vi "绘制语法框.vi"(8 "error in":errorcluster caption="错误输入（无错误）", 11 "程序 输入":refnum<class "程序.lvclass">) -> (0 "error out":errorcluster caption="错误输出", 3 "程序 输出":refnum<class "程序.lvclass">)   [LabVIEW 2020, in "程序.lvclass"]
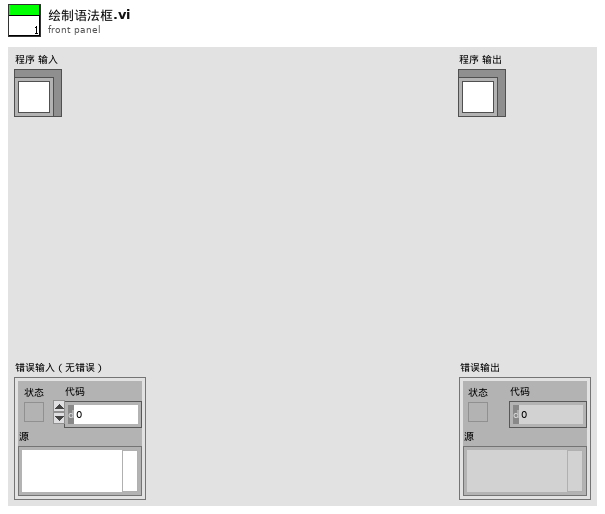
[diagram p1: front panel]
types:
  T1 = cluster{"left":i16, "top":i16, "right":i16, "bottom":i16}
  T2 = cluster{"Width":i16, "Style":enum32{"Solid", "Dash", "Dot", "DashDot", "DashDotDot"}}
  T3 = typedef "LVBoundsTypeDef.ctl" = cluster{"Width":u32, "Height":u32}
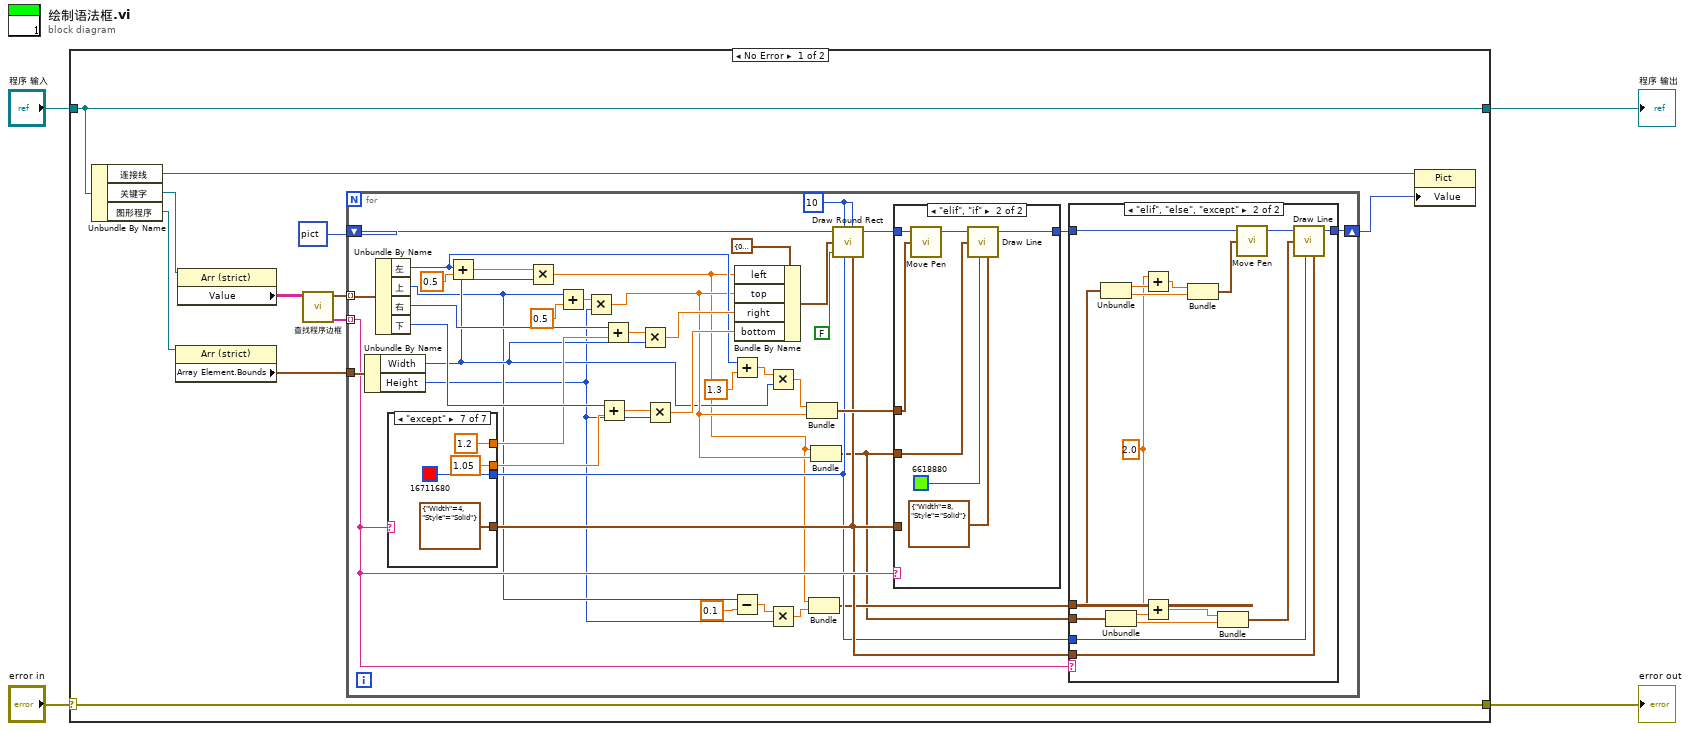
[diagram p0: block diagram]
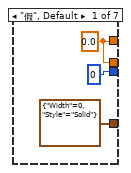
[diagram p4: hidden frame]
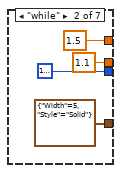
[diagram p5: hidden frame]
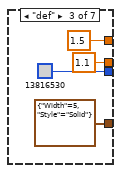
[diagram p6: hidden frame]
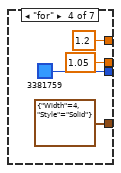
[diagram p7: hidden frame]
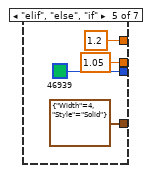
[diagram p8: hidden frame]
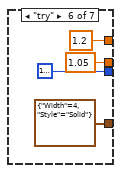
[diagram p9: hidden frame]
diagram:
  n1 = case shown="No Error" "error in" {
    selector: "error in" -> [w15 w109]
    tunnel: [w15 w109] -> w3
    tunnel: [w14 w108] -> w1
    tunnel: "程序 输入" -> [w14 w108]
    frame No Error {
      n2 = Unbundle By Name(w14) -> ("连接线"=w7:refnum<vi>, "关键字"=w13:refnum<vi>, "图形程序"=w10:refnum<vi>)
      n3 = property class="Arr (strict)"(reference=w10) -> ("Array Element.Bounds"=w8:T3)  [unwired: 1 in, 2 out]
      n4 = property class="Arr (strict)"(reference=w13) -> ("Value"=w12:string[][])  [unwired: 1 in, 2 out]
      n5 = call "查找程序边框.vi"("数组"=w12) -> ("类型"=w5:string[], "边界"=w9:cluster{"左":i32, "上":i32, "右":i32, "下":i32}[])  [unwired: 9 in]
      n6 = for {
        shift-right: [w29] -> w6
        shift-left: picture data[5B] ("picture") -> [w55]
        tunnel: w9 -> [w54] mode=indexing
        tunnel: w8 -> [w53]
        tunnel: w5 -> [w28] mode=indexing
        w40 = i16 10 ("oval width")
        n7 = Unbundle By Name(w53) -> ("Width"=w22:u32, "Height"=w19:u32)
        n8 = Unbundle By Name(w54) -> ("左"=w37:i32, "上"=w20:i32, "右"=w44:i32, "下"=w42:i32)
        n9 = case shown="\"except\"" w28 {
          tunnel: [T2 {"Width"=0, "Style"=enum."Solid"} ("pen") T2 {"Width"=5, "Style"=enum."Solid"} ("pen") T2 {"Width"=5, "Style"=enum."Solid"} ("pen") T2 {"Width"=4, "Style"=enum."Solid"} ("pen") T2 {"Width"=4, "Style"=enum."Solid"} ("pen") T2 {"Width"=4, "Style"=enum."Solid"} ("pen") T2 {"Width"=4, "Style"=enum."Solid"} ("pen")] -> w27
          tunnel: [u32 0 ("color(black)") u32 16777222 ("color(black)") u32 13816530 ("color(black)") u32 3381759 ("color(black)") u32 46939 ("color(black)") u32 16777224 ("color(black)") u32 16711680 ("color(black)")] -> w26
          tunnel: [w81 1.5 1.5 1.2 1.2 1.2 1.2] -> w39
          tunnel: [w81 1.1 1.1 1.05 1.05 1.05 1.05] -> w31
          frame "假", Default {
            w81 = 0.0
          }
          frame "while" {
          }
          frame "def" {
          }
          frame "for" {
          }
          frame "elif", "else", "if" {
          }
          frame "try" {
          }
          frame "except" {
          }
        }
        n10 = Add(x=w37, y=0.5) -> (x+y=w51:dbl)
        n11 = Multiply(x=w51, y=w22) -> (x*y=w18:dbl)
        n12 = Add(x=w20, y=0.5) -> (x+y=w50:dbl)
        n13 = Multiply(x=w50, y=w19) -> (x*y=w32:dbl)
        n14 = Add(x=w42, y=w31) -> (x+y=w41:dbl)
        n15 = Add(x=w44, y=w39) -> (x+y=w43:dbl)
        n16 = Multiply(x=w43, y=w22) -> (x*y=w47:dbl)
        n17 = Multiply(x=w41, y=w19) -> (x*y=w46:dbl)
        n18 = Add(x=w37, y=1.3) -> (x+y=w35:dbl)
        n19 = Subtract(x=w20, y=0.1) -> (x-y=w24:dbl)
        n20 = Bundle By Name(cluster=T1 {"left"=0, "top"=0, "right"=0, "bottom"=0} ("rect"), "left"=w18, "top"=w32, "right"=w47, "bottom"=w46) -> (w45:T1)
        n21 = Multiply(x=w35, y=w22) -> (x*y=w34:dbl)
        n22 = Multiply(x=w24, y=w19) -> (x*y=w21:dbl)
        n23 = Bundle(w34, w32) -> (w33:cluster{dbl, dbl})  [unwired: 1 in]
        n24 = Bundle(w18, w21) -> (w25:cluster{dbl, dbl})  [unwired: 1 in]
        n25 = Bundle(w18, w32) -> (w17:cluster{dbl, dbl})  [unwired: 1 in]
        n26 = call <vilib>:"Draw Round Rect.vi"("picture"=w55, "oval width"=w40, "rect"=w45, "fill?(F)"=FALSE, "color(black)"=w26, "oval height"=w40, "pen"=w27) -> ("new picture"=w38:picture)  [unwired: 2 in]
        n27 = case shown="\"elif\", \"if\"" w28 {
          tunnel: w38 -> [w73 w80]
          tunnel: [w73 w77] -> w30
          tunnel: w33 -> [_ w78]
          tunnel: w17 -> [_ w76]
          tunnel: w27 -> [_ _]
          frame "假", Default {
          }
          frame "elif", "if" {
            n28 = call <vilib>:"Move Pen.vi"("new position"=w78, "picture"=w80) -> ("new picture"=w79:picture)  [unwired: 3 in]
            n29 = call <vilib>:"Draw Line.vi"("picture"=w79, "end point"=w76, "color(black)"=u32 6618880, "pen"=T2 {"Width"=8, "Style"=enum."Solid"}) -> ("new picture"=w77:picture)  [unwired: 5 in]
          }
        }
        n30 = case shown="\"elif\", \"else\", \"except\"" w28 {
          tunnel: w30 -> [w56 w72]
          tunnel: [w56 w70] -> w29
          tunnel: w25 -> [_ w67]
          tunnel: w17 -> [_ w63]
          tunnel: w26 -> [_ w69]
          tunnel: w27 -> [_ w68]
          frame "假", Default {
          }
          frame "elif", "else", "except" {
            w57 = 2.0 ("y")
            n31 = Unbundle(w67) -> (w61:dbl, w66:dbl)
            n32 = Unbundle(w63) -> (w58:dbl, w64:dbl)
            n33 = Add(x=w57, y=w61) -> (x+y=w60:dbl)
            n34 = Add(x=w57, y=w58) -> (x+y=w59:dbl)
            n35 = Bundle(w60, w66) -> (w65:cluster{dbl, dbl})  [unwired: 1 in]
            n36 = Bundle(w59, w64) -> (w62:cluster{dbl, dbl})  [unwired: 1 in]
            n37 = call <vilib>:"Move Pen.vi"("new position"=w65, "picture"=w72) -> ("new picture"=w71:picture)  [unwired: 3 in]
            n38 = call <vilib>:"Draw Line.vi"("picture"=w71, "end point"=w62, "color(black)"=w69, "pen"=w68) -> ("new picture"=w70:picture)  [unwired: 5 in]
          }
        }
      }
      n39 = property class="Pict"(reference=w7, "Value"=w6) -> ()  [unwired: 1 in, 2 out]
    }
    frame Error {
    }
  }
  "error out" <- w3
  "程序 输出" <- w1
